vi "axis_Grab.vi"() -> ()   [LabVIEW 2009]
panel:
  in  "Color?":bool=TRUE
  in  "Pixel Format":T1(ring)
  out "error out":errorcluster={"status"=TRUE, "code"=-1074396120, "source"="IMAQ ReadFile\n  Not an image."}
  out "Content Length":i32=37577
  in  "stop":bool
  in  "Frame Rate":u32(slide) max=30 scale=0.0..30.0
  out "Image":T2(plugin-control)
  in  "address":string="10.0.58.10"
  in  "Compression":u32(slide)=25 scale=0.0..99.0
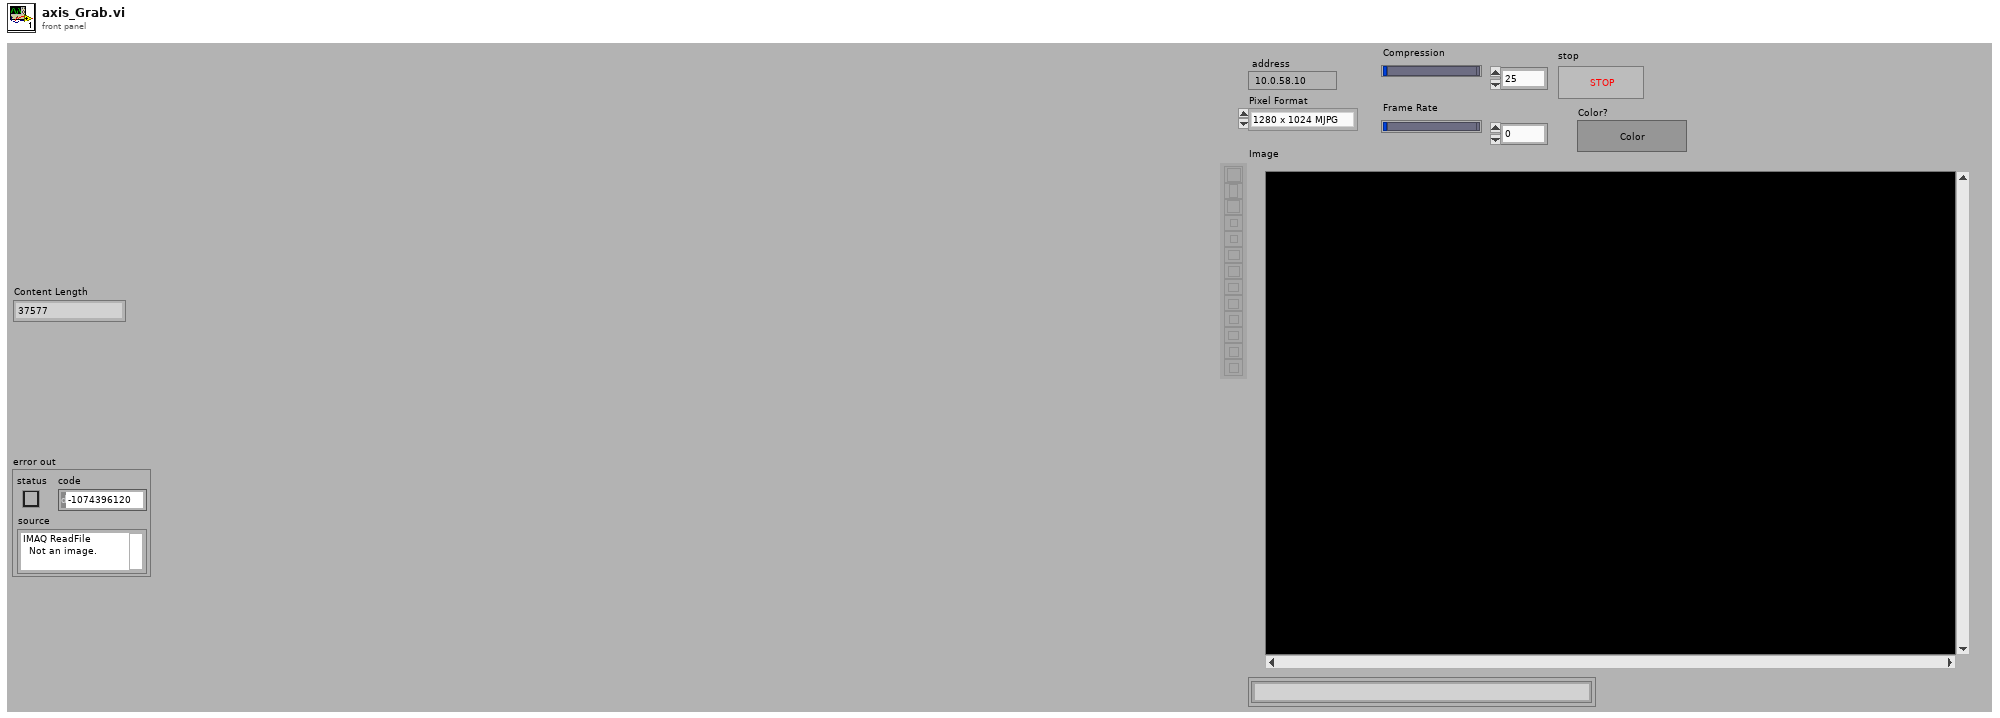
[diagram p1: front panel]
types:
  T1 = enum16{"1280 x 1024 MJPG", "1280 x 960 MJPG", "1280 x 720 MJPG", "1280 x 480 MJPG", "640 x 480 MJPG", "320 x 240 MJPG", "160 x 120 MJPG"}
  T2 = typedef "IMAQ Image.ctl" = refnum<image>
  T3 = enum16{"Standard", "Buffered", "CRLF", "Immediate"}
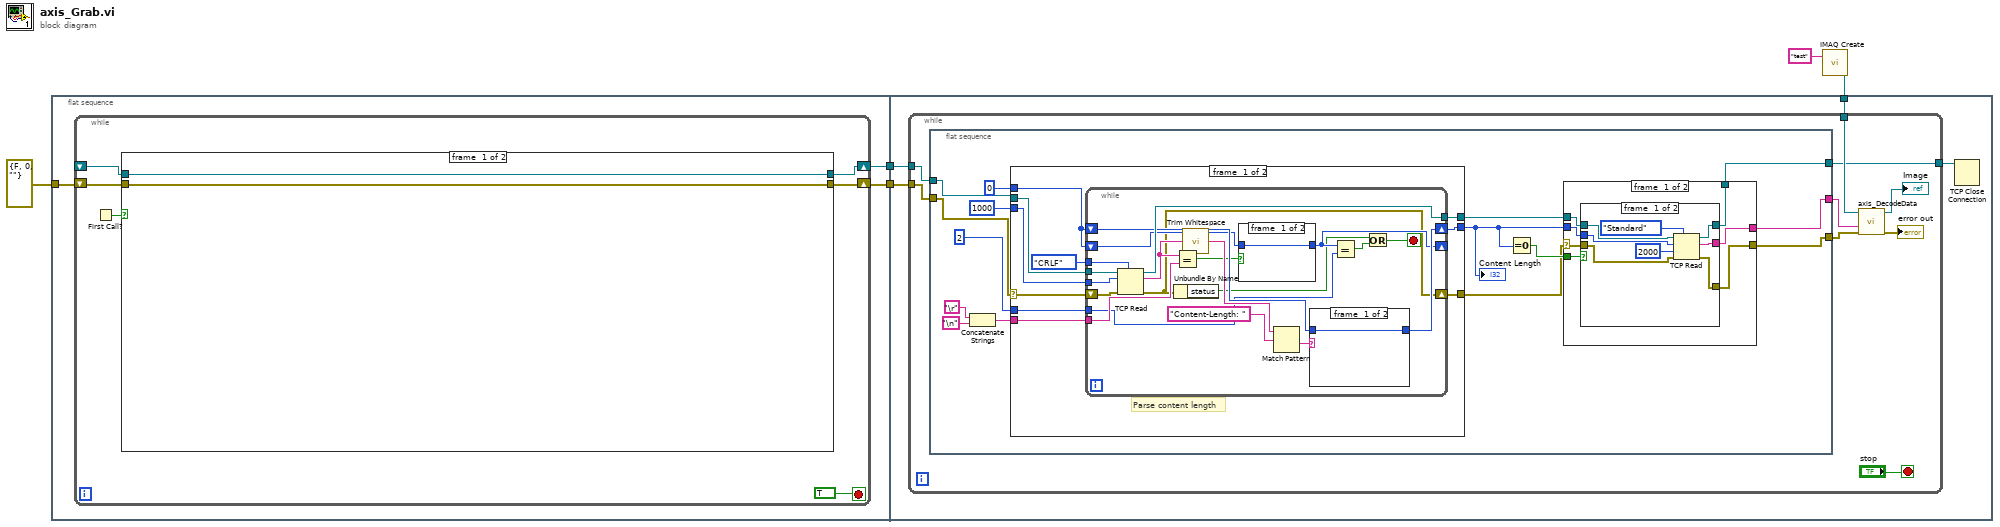
[diagram p0: block diagram]
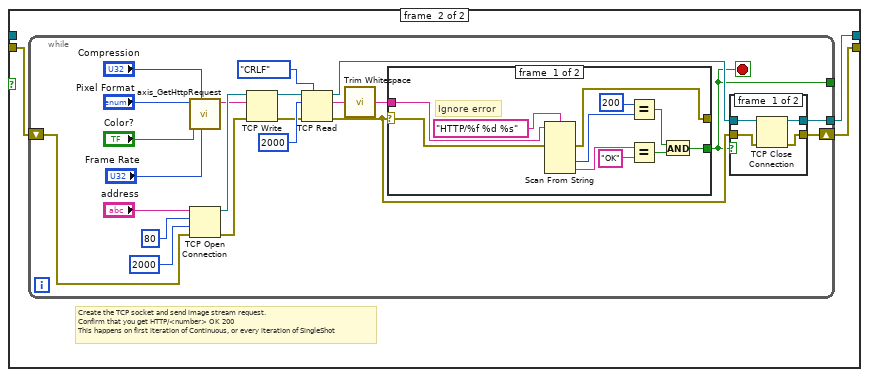
[diagram p2: hidden frame]
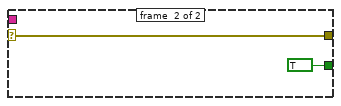
[diagram p4: hidden frame]
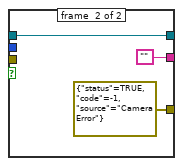
[diagram p5: hidden frame]
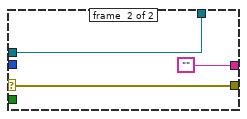
[diagram p6: hidden frame]
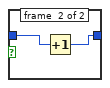
[diagram p7: hidden frame]
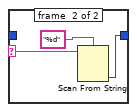
[diagram p8: hidden frame]
diagram:
  n1 = flat-sequence {
    tunnel: errorcluster {"status"=FALSE, "code"=0, "source"=""} ("error out") -> [w8]
    tunnel: [w7] -> w3
    tunnel: [w6] -> w2
    tunnel: w3 -> [w64]
    tunnel: w2 -> [w63]
    tunnel: w1 -> [w62]
    frame #0 {
      n2 = while {
        shift-right: [w11] -> w7
        shift-left: _ -> [w10]
        shift-right: [w12] -> w6
        shift-left: w8 -> [w13]
        stop <- TRUE stop-if-true
        n3 = First Call?() -> (First Call?: T/F=w9:bool)
        n4 = case shown="True" w9 {
          tunnel: w13 -> [w15 w19]
          tunnel: [w15 w18] -> w12
          tunnel: [w16 w17] -> w11
          tunnel: w10 -> [w16 _]
          frame #0 {
          }
          frame #1 {
            # "Create the TCP socket and send image stream request.\nConfirm that you get HTTP/<number> OK 200\nThis happens on first iteration of Continuous, or every iteration of SingleShot"
            n5 = while {
              shift-right: [w27] -> w18
              shift-left: w19 -> [w32]
              tunnel: [w26] -> _
              tunnel: [w28] -> w17
              stop <- w26 stop-if-true
              n6 = call "axis_GetHttpRequest.vi"("Frame Rate"="Frame Rate", "Compression"="Compression", "Color?"="Color?", "Pixel Format"="Pixel Format") -> ("HTTP Request"=w25:string)  [unwired: 7 out]
              n7 = TCP Open Connection(address="address", remote port or service name=u16 80, timeout ms (60000)=2000, error in (no error)=w32) -> (connection ID=w33:refnum<k5>, error out=w31:errorcluster)  [unwired: 1 out]
              n8 = TCP Write(connection ID=w33, data in=w25, error in (no error)=w31) -> (connection ID out=w37:refnum<k5>, error out=w36:errorcluster)  [unwired: 2 out]
              n9 = TCP Read(connection ID=w37, bytes to read=2000, error in (no error)=w36, 7:T3."CRLF" ("mode (standard)")) -> (connection ID out=w30:refnum<k5>, data out=w41:string, error out=w29:errorcluster)  [unwired: 1 out]
              n10 = call <vilib>:"Trim Whitespace.vi"("string"=w41) -> ("trimmed string"=w39:string)  [unwired: 1 in]
              n11 = case shown="No Error" w29 {
                selector: w29 -> [w49 w60]
                tunnel: w39 -> [w58 _]
                tunnel: [w50 TRUE] -> w26
                tunnel: [w48 w60] -> _
                frame #0 {
                  # "Ignore error"
                  n12 = Scan From String(format string="HTTP/%f %d %s", input string=w58, error in=w49) -> (error out=w48:errorcluster, output 2=w56:i32, output 3=w54:string)  [unwired: 1 in, 6 out]
                  n13 = Equal?(x=200, y=w56) -> (x = y?=w51:bool)
                  n14 = Equal?(x=w54, y="OK" ("format string")) -> (x = y?=w52:bool)
                  n15 = And(x=w51, y=w52) -> (x .and. y?=w50:bool)
                }
                frame #1 {
                }
              }
              n16 = case shown="False" w26 {
                tunnel: w30 -> [w45 w47]
                tunnel: w29 -> [w44 w46]
                tunnel: [w43 w47] -> w28
                tunnel: [w42 w46] -> w27
                frame #0 {
                  n17 = TCP Close Connection(connection ID=w45, error in (no error)=w44) -> (connection ID out=w43:refnum<k5>, error out=w42:errorcluster)  [unwired: 1 out]
                }
                frame #1 {
                }
              }
            }
          }
        }
      }
    }
    frame #1 {
      n18 = while {
        tunnel: w64 -> [w73]
        tunnel: w63 -> [w72]
        tunnel: w62 -> [w69]
        tunnel: [w65] -> w61
        stop <- "stop" stop-if-true
        n19 = flat-sequence {
          tunnel: w72 -> [w80]
          tunnel: [w77] -> w67
          tunnel: [w79] -> w68
          tunnel: w73 -> [w78]
          tunnel: [w74] -> w65
          frame #0 {
            n20 = Concatenate Strings("\r", "\n") -> (w88:string)
            n21 = case shown="No Error" w80 {
              selector: w80 -> [w112 w148]
              tunnel: [w119 w148] -> w83
              tunnel: [w118 w149] -> w85
              tunnel: [w117 w147] -> w75
              tunnel: w88 -> [w116 _]
              tunnel: 0 -> [w115 w149]
              tunnel: 1000 ("bytes to read") -> [w113 _]
              tunnel: w78 -> [w111 w147]
              tunnel: 2 ("y") -> [w110 _]
              frame #0 {
                # "Parse content length"
                n22 = while {
                  tunnel: [w139] -> w117
                  shift-right: [w135] -> w118
                  shift-left: w115 -> [w134]
                  shift-right: [w131] -> _
                  shift-left: w115 -> [w132]
                  tunnel: w116 -> [w129]
                  tunnel: w113 -> [w128]
                  tunnel: T3."CRLF" ("mode (standard)") -> [w127]
                  shift-right: [w125] -> w119
                  shift-left: w112 -> [w126]
                  tunnel: w111 -> [w121]
                  tunnel: w110 -> [w120]
                  stop <- w122 stop-if-true
                  n23 = TCP Read(connection ID=w121, bytes to read=w128, error in (no error)=w126, 7:w127) -> (connection ID out=w139:refnum<k5>, data out=w130:string, error out=w125:errorcluster)  [unwired: 1 out]
                  n24 = Unbundle By Name(w125) -> ("status"=w124:bool)
                  n25 = Equal?(x=w130, y=w129) -> (x = y?=w133:bool)
                  n26 = call <vilib>:"Trim Whitespace.vi"("string"=w130) -> ("trimmed string"=w137:string)  [unwired: 1 in]
                  n27 = case shown="True" w133 {
                    tunnel: w132 -> [w140 w142]
                    tunnel: [w140 w141] -> w131
                    frame #0 {
                    }
                    frame #1 {
                      n28 = Increment(x=w142) -> (x+1=w141:i32)
                    }
                  }
                  n29 = Match Pattern(string=w137, regular expression="Content-Length: ") -> (after substring=w136:string)  [unwired: 4 out]
                  n30 = case shown="\"True\", Default" w136 {
                    selector: w136 -> [_ w145]
                    tunnel: [w143 w146] -> w135
                    tunnel: w134 -> [w143 _]
                    frame #0 {
                    }
                    frame #1 {
                      n31 = Scan From String(format string="%d", input string=w145) -> (output 1=w146:i32)  [unwired: 2 in, 4 out]
                    }
                  }
                  n32 = Equal?(x=w131, y=w120) -> (x = y?=w123:bool)
                  n33 = Or(x=w124, y=w123) -> (x .or. y?=w122:bool)
                }
              }
              frame #1 {
              }
            }
            "Content Length" <- w85
            n34 = Equal To 0?(x=w85) -> (x = 0?=w86:bool)
            n35 = case shown="No Error" w83 {
              selector: w83 -> [w90 w109]
              tunnel: [w95 w109] -> w77
              tunnel: [w94 ""] -> w79
              tunnel: w86 -> [w93 _]
              tunnel: w85 -> [w92 _]
              tunnel: w75 -> [w91 w107]
              tunnel: [w89 w107] -> w74
              frame #0 {
                n36 = case shown="False" w93 {
                  tunnel: w91 -> [w103 w105]
                  tunnel: [w102 errorcluster {"status"=TRUE, "code"=-1, "source"="Camera Error"} ("error out")] -> w95
                  tunnel: [w98 ""] -> w94
                  tunnel: w92 -> [w99 _]
                  tunnel: [w97 w105] -> w89
                  tunnel: w90 -> [w96 _]
                  frame #0 {
                    n37 = TCP Read(connection ID=w103, bytes to read=w99, error in (no error)=w96, 7:T3."Standard" ("mode (standard)"), 9:2000 ("timeout ms (25000)")) -> (connection ID out=w97:refnum<k5>, data out=w98:string, error out=w102:errorcluster)
                  }
                  frame #1 {
                  }
                }
              }
              frame #1 {
              }
            }
          }
        }
        n38 = call "axis_DecodeData.vi"("error IO"=w67, "Data In"=w68, "Image In"=w69) -> ("error out"=→"error out":errorcluster, "Image Out"=→"Image":T2)  [unwired: 1 in, 6 out]
      }
      n39 = TCP Close Connection(connection ID=w61) -> ()  [unwired: 2 in, 2 out]
    }
  }
  n40 = call "IMAQ Create"("Image Name"="test") -> ("New Image"=w1:T2)  [unwired: 3 in, 2 out]
